vi "Задание_АБ_правильное_детектирование.vi"() -> ()   [LabVIEW 2017]
uses:
  <vilib>/Analysis/baseanly.llb/Mean (DBL).vi
  <vilib>/gmath/statdist.llb/Beta Random.vi
  <vilib>/Analysis/3filter.llb/Bessel Filter (DBL).vi
  <vilib>/Analysis/NI_AALBase.lvlib
  <vilib>/gmath/NI_Gmath.lvlib
panel:
  out "Демодулированный сигнал 2":i16[](graph)
  out "0, 1":i16[](array[numeric])
  in  "Пороговое значение 2":dbl
  out "x/y":dbl
  out "Среднее значение":dbl[](array[numeric])
  out "Шум на основе распределения Рэлея":dbl[](graph)
  out "Итого. кол-во бит":i32
  in  "Пороговое значение":dbl
  out "Демодулированный и отфильтрованный сигнал":dbl[](graph)
  out "Демодулированный сигнал":i16[](graph)
  in  "Нижняя частота среза":dbl
  in  "Порядок фильтра":i64(slide) scale=0.0..20.0
  in  "Переменная floor(x/y)":i32
  out "Модулирующий сигнал":dbl[](graph)
  out "Частотно модулированный цифровой сигнал":dbl[](graph)
  in  "см. 1.2 Циклов в секунду":i32(slide) scale=4.0..50.0
  in  "Сколько битов брать":i32=4
  out "Радио сигнал с паузами":dbl[](graph)
  in  "Кол-во выборок":i32=400
  out "Массив с паузами":dbl[](array[numeric])
  in  "Количество бит":i32=8
  out "Вырезка из массива":dbl[](array[numeric])
  out "Биты на выходе 1":dbl[](array[numeric])
  # "Демодуляция"
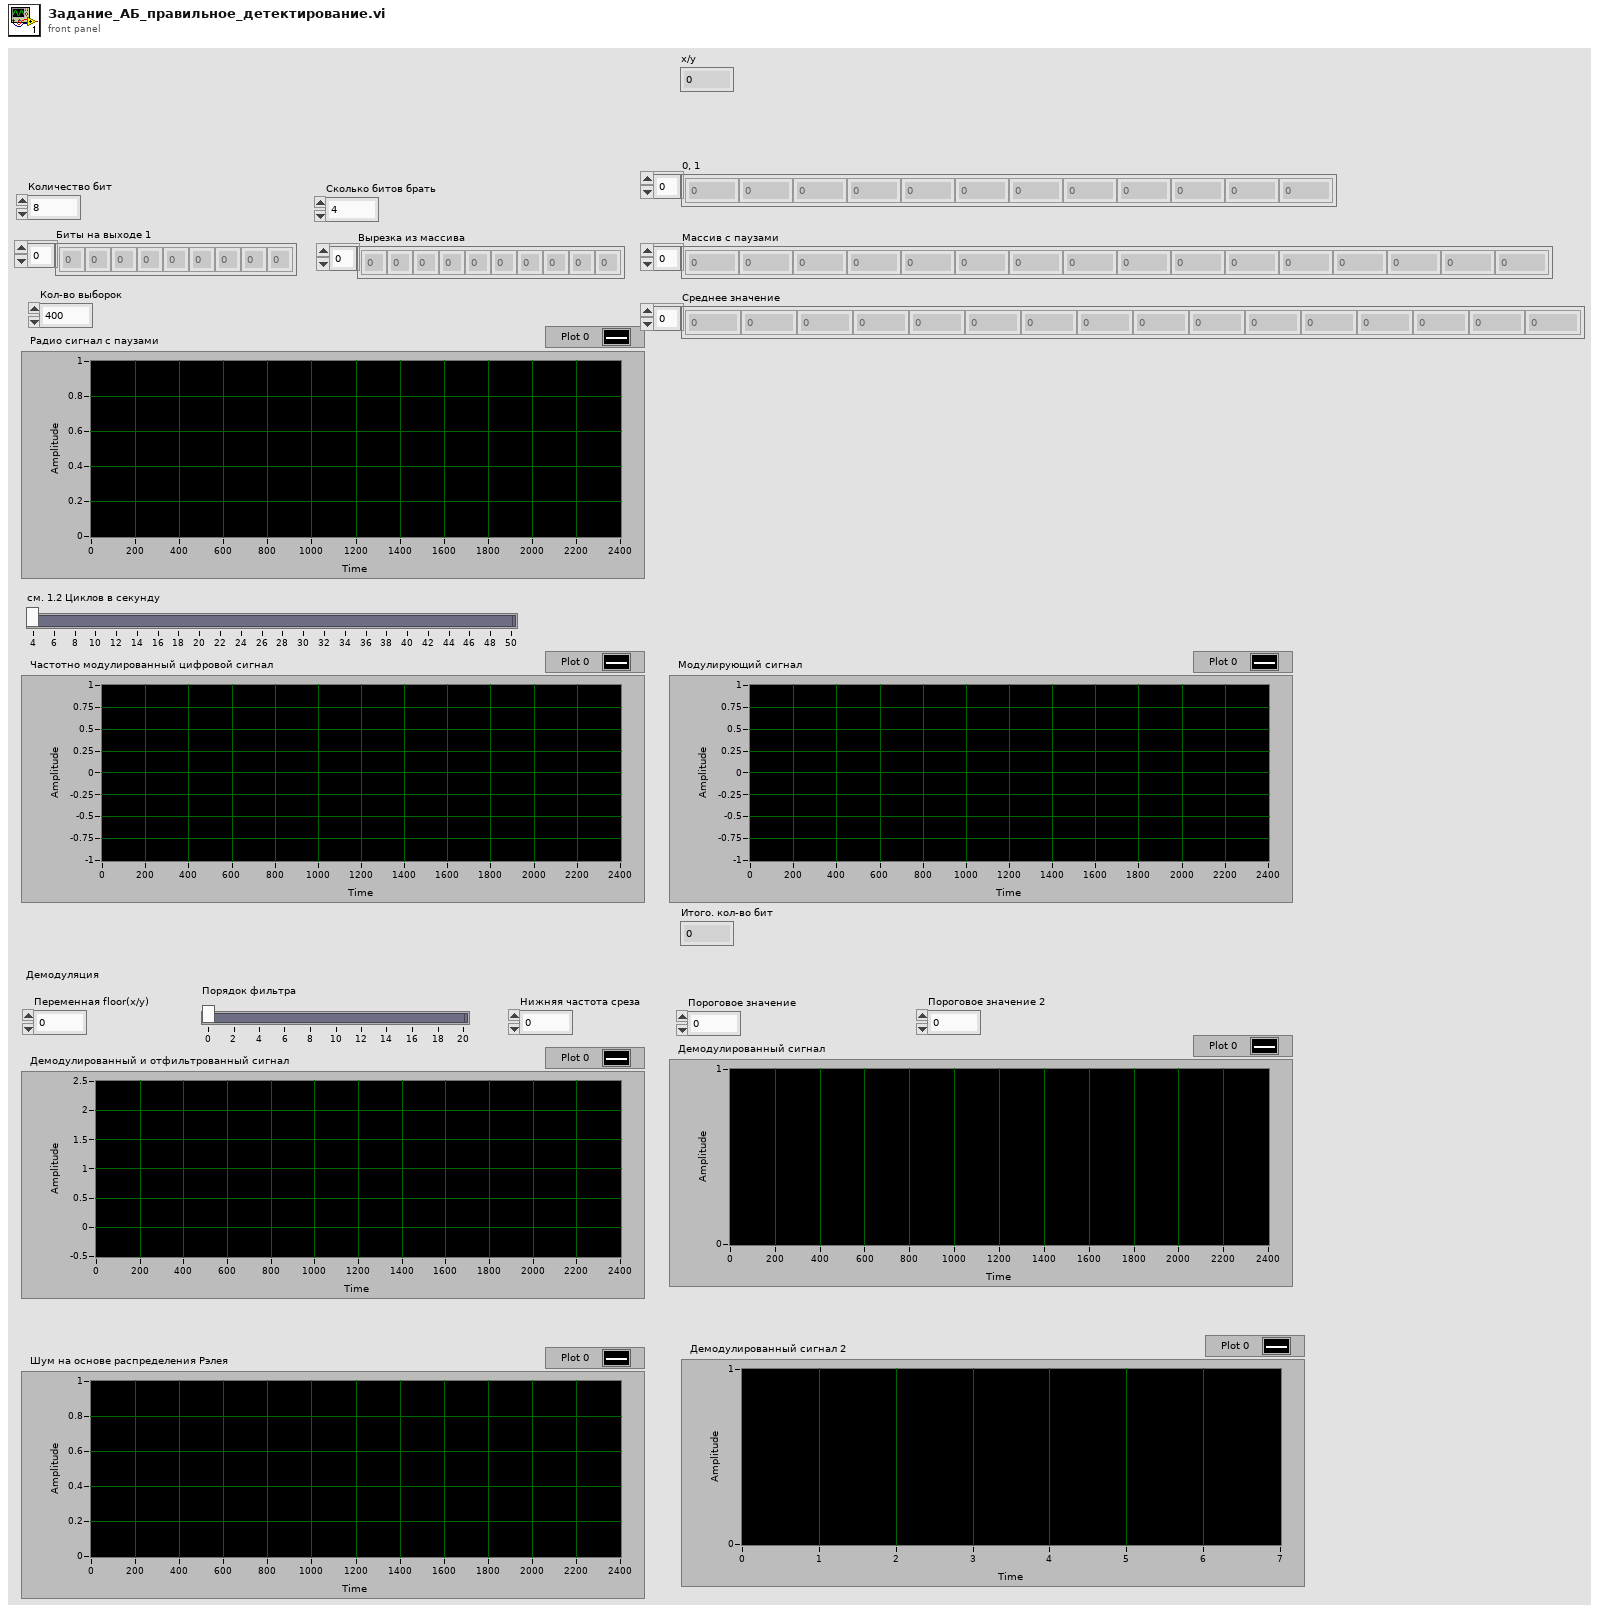
[diagram p1: front panel]
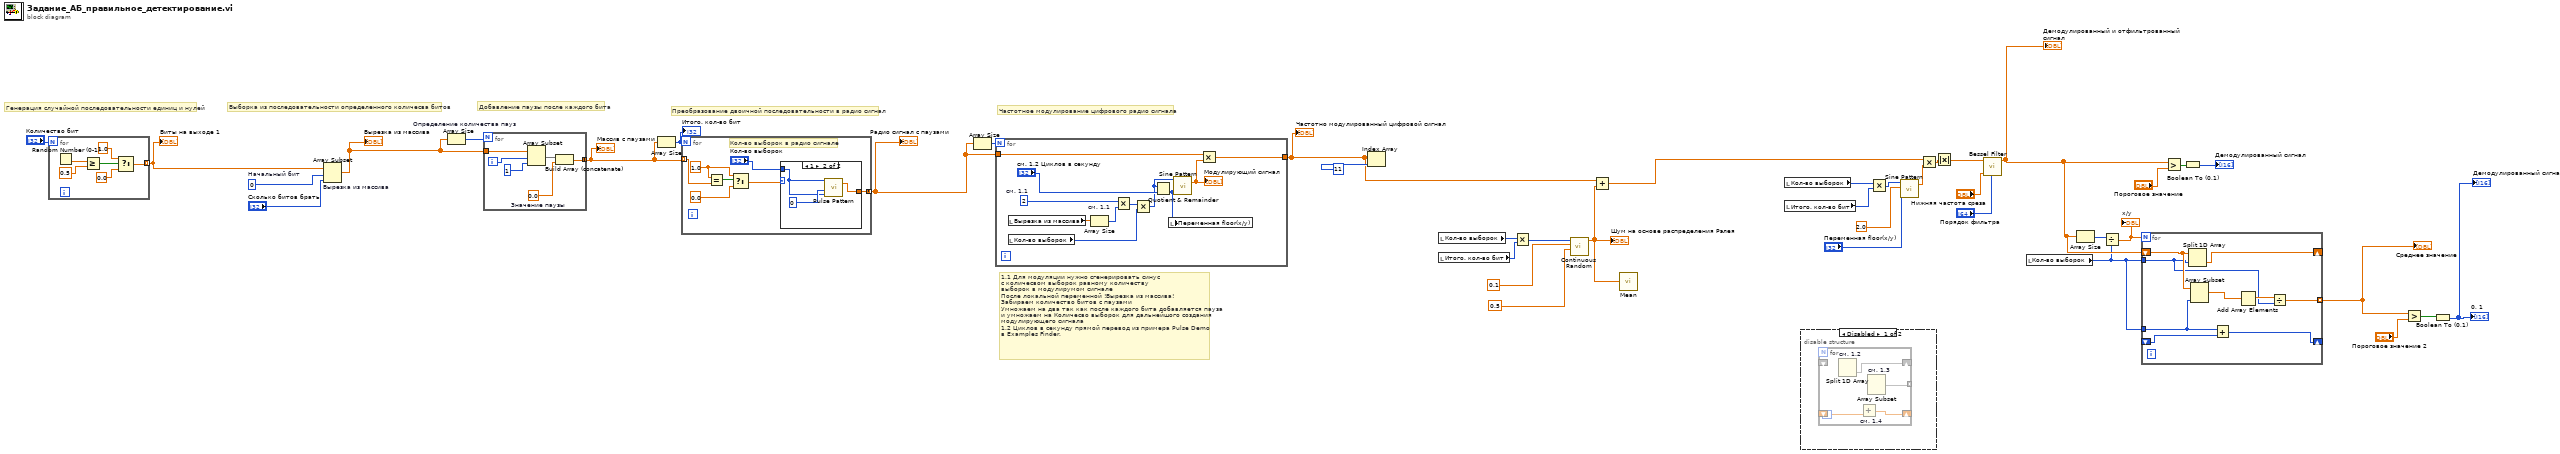
[diagram p0: block diagram]
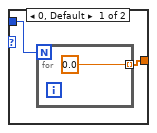
[diagram p3: hidden frame]
diagram:
  w39 = 0  # Начальный бит
  # "1.1 Для модуляции нужно сгенерировать синус \nс количесвом выборок равному количеству \nвыборок в модулирумом сигнале\nПосле локальной переменной !Вырезка из массива! \nЗабираем количество битов с паузами \nУмножаем на два так как после каждого бита добавляется пауза\nи умножаем на Количесво выборок для дальнейшого создания  \nмодулирующего сигнала\n1.2 Циклов в секунду прямой перевод из примера Pulse Demo \nв Examples Finder."
  # "Преобразование двоичной последовательности в радио сигнал"
  # "Частотное модулирование цифрового радио сигнала"
  # "Добавление паузы после каждого бита"
  # "Выборка из последовательности определенного количесва битов"
  # "Генерация случайной последовательности единиц и нулей"
  n1 = for {
    N: "Количество бит" -> [_]
    tunnel: [w41] -> w37 mode=indexing
    n2 = Random Number (0-1)() -> (number: 0 to 1=w46:dbl)
    n3 = Greater Or Equal?(x=w46, y=0.5) -> (x >= y?=w44:bool)
    n4 = Select(t=1.0, s=w44, f=0.0) -> (s? t:f=w41:dbl)
  }
  "Биты на выходе 1" <- w37
  n5 = Array Subset "Вырезка из массива"(array=w37, index=w39, length="Сколько битов брать") -> (w35:dbl[])
  "Вырезка из массива" <- w35
  n6 = Array Size "Определение количества пауз"(array=w35) -> (size(s)=w36:i32)
  n7 = for {
    N: w36 -> [_]
    tunnel: w35 -> [w49]
    tunnel: [w48] -> w32 mode=concatenating
    i -> [w47]
    w50 = 0.0  # Значение паузы
    n8 = Array Subset(array=w49, index=w47, length=1) -> (w51:dbl[])
    n9 = Build Array (concatenate)(w51, w50) -> (w48:dbl[])
  }
  "Массив с паузами" <- w32
  n10 = Array Size(array=w32) -> (size(s)=w33:i32)
  "Итого. кол-во бит" <- w33
  n11 = for {
    N: w33 -> [_]
    tunnel: w32 -> [w56] mode=indexing
    tunnel: [w54] -> w31 mode=concatenating
    w58 = 1.0
    # "Кол-во выборок в радио сигнале"
    n12 = Equal?(x=w58, y=w56) -> (x = y?=w59:bool)
    n13 = Select(t=w58, s=w59, f=0.0) -> (s? t:f=w55:dbl)
    n14 = case shown="1" w55 {
      tunnel: [w60 w64] -> w54
      tunnel: "Кол-во выборок" -> [w61 w63]
      frame 0, Default {
        n15 = for {
          N: w61 -> [_]
          tunnel: [0.0] -> w60 mode=indexing
        }
      }
      frame 1 {
        n16 = call <vilib>:"Pulse Pattern.vi"("width"=w63, "delay"=0, "samples"=w63) -> ("Pulse Pattern"=w64:dbl[])  [unwired: 1 in, 1 out]
      }
    }
  }
  "Радио сигнал с паузами" <- w31
  n17 = Array Size(array=w31) -> (size(s)=w34:i32)
  n18 = for {
    N: w34 -> [_]
    tunnel: w31 -> [w75]
    tunnel: [w74] -> w10
    w70 = 2  # см. 1.1
    n19 = local read "Вырезка из массива"() -> (w72:dbl[])
    n20 = local read "Кол-во выборок"() -> (w68:i32)
    n21 = Array Size "см. 1.1"(array=w72) -> (size(s)=w71:i32)
    n22 = Multiply(x=w70, y=w71) -> (x*y=w69:i32)
    n23 = Multiply(x=w69, y=w68) -> (x*y=w67:i32)
    n24 = Quotient & Remainder(x=w67, y="см. 1.2 Циклов в секунду") -> (floor(x/y)=w66:i32)  [unwired: 1 out]
    n25 = local write "Переменная floor(x/y)"(w66) -> ()
    n26 = call <vilib>:"Sine Pattern.vi"("cycles"=w66, "samples"=w67) -> ("Sinusoidal Pattern"=w73:dbl[])  [unwired: 2 in, 1 out]
    "Модулирующий сигнал" <- w73
    n27 = Multiply(x=w75, y=w73) -> (x*y=w74:dbl[])
  }
  "Частотно модулированный цифровой сигнал" <- w10
  n28 = Index Array(array=w10, index=11 ("index (row)")) -> ()  [unwired: 1 out]
  n29 = local read "Кол-во выборок"() -> (w14:i32)
  n30 = local read "Итого. кол-во бит"() -> (w13:i32)
  n31 = Multiply(x=w14, y=w13) -> (x*y=w12:i32)
  n32 = call-poly <vilib>:"Continuous Random.vi"("b"=0.5, "a"=0.1 ("x"), "samples"=w12) -> ("beta random data"=w11:dbl[])  [unwired: 7 in, 1 out]
  "Шум на основе распределения Рэлея" <- w11
  n33 = Add(x=w10, y=w11) -> (x+y=w9:dbl[])
  n34 = call-poly <vilib>:"Mean.vi"("X"=w11) -> ()  [unwired: 2 out]
  n35 = local read "Кол-во выборок"() -> (w18:i32)
  n36 = local read "Итого. кол-во бит"() -> (w17:i32)
  n37 = disable-structure shown="Disabled" {
    frame Disabled {
      n38 = for {
        shift-right: [w80] -> _
        shift-left: _ -> [_]
        shift-right: [w79] -> _
        shift-left: _ -> [w78]
        tunnel: [w77] -> _ mode=indexing
        n39 = Split 1D Array "см. 1.2"() -> (second subarray=w80:void[])  [unwired: 2 in, 1 out]
        n40 = Add "см. 1.4"(y=w78) -> (x+y=w79:dbl)  [unwired: 1 in]
        n41 = Array Subset "см. 1.3"() -> (w77:void[])  [unwired: 3 in]
      }
    }
    frame Enabled {
    }
  }
  n42 = Multiply(x=w18, y=w17) -> (x*y=w19:i32)
  n43 = call <vilib>:"Sine Pattern.vi"("cycles"="Переменная floor(x/y)", "amplitude"=2.0, "samples"=w19) -> ("Sinusoidal Pattern"=w20:dbl[])  [unwired: 1 in, 1 out]
  n44 = Multiply(x=w9, y=w20) -> (x*y=w27:dbl[])
  n45 = Absolute Value(x=w27) -> (abs(x)=w24:dbl[])
  n46 = call-poly <vilib>:"Bessel Filter.vi"("order"="Порядок фильтра", "low cutoff freq: fl"="Нижняя частота среза", "X"=w24) -> ("Filtered X"=w7:dbl[])  [unwired: 5 in, 1 out]
  "Демодулированный и отфильтрованный сигнал" <- w7
  n47 = local read "Кол-во выборок"() -> (w6:i32)
  n48 = Array Size(array=w7) -> (size(s)=w8:i32)
  n49 = Divide(x=w8, y=w6) -> (x/y=w5:dbl)
  "x/y" <- w5
  n50 = for {
    N: w5 -> [_]
    tunnel: w6 -> [w82]
    shift-right: [w89] -> _
    shift-left: w7 -> [w88]
    tunnel: w6 -> [w85]
    shift-right: [w86] -> _
    shift-left: _ -> [w87]
    tunnel: [w81] -> w3 mode=indexing
    n51 = Split 1D Array(array=w88, index=w82) -> (second subarray=w89:dbl[])  [unwired: 1 out]
    n52 = Array Subset(array=w88, length=w85) -> (w84:dbl[])  [unwired: 1 in]
    n53 = Add(x=w85, y=w87) -> (x+y=w86:i32)
    n54 = Add Array Elements(numeric array=w84) -> (sum=w83:dbl)
    n55 = Divide(x=w83, y=w82) -> (x/y=w81:dbl)
  }
  "Среднее значение" <- w3
  n56 = Greater?(x=w7, y="Пороговое значение") -> (0:w23:bool[])
  n57 = Boolean To (0,1)(Boolean=w23) -> (0, 1=→"Демодулированный сигнал":i16[])
  n58 = Greater?(x=w3, y="Пороговое значение 2") -> (0:w2:bool[])
  n59 = Boolean To (0,1)(Boolean=w2) -> (0, 1=→"0, 1" →"Демодулированный сигнал 2":i16[])
